vi "Material-PassFail-LineN.vi"(8 "error in (no error)":errorcluster, 10 "Line?":i32, 11 "Material-RunTest in":refnum<class "Material-RunTest.lvclass">) -> (0 "error out":errorcluster, 3 "Material-RunTest out":refnum<class "Material-RunTest.lvclass">)   [LabVIEW 2013, in "Material-RunTest.lvclass"]
uses:
  Material-RunTest.lvclass
  Material-RunTest.lvclass/Material-RunTest.ctl
  <userlib>/_MGI/1D Array/MGI Average/MGI Average (DBL[]).vi
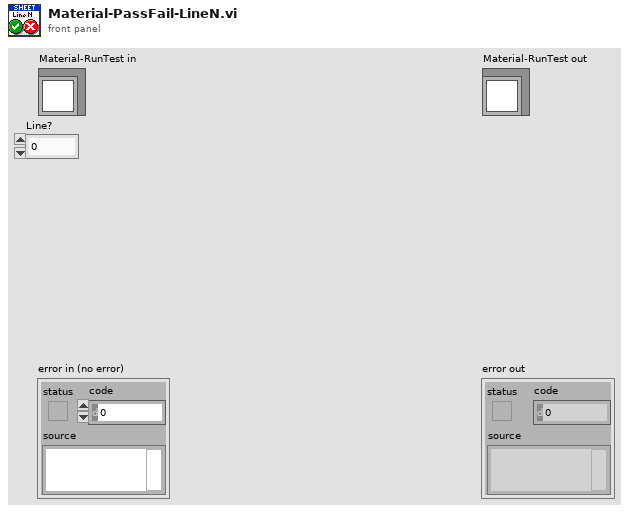
[diagram p1: front panel]
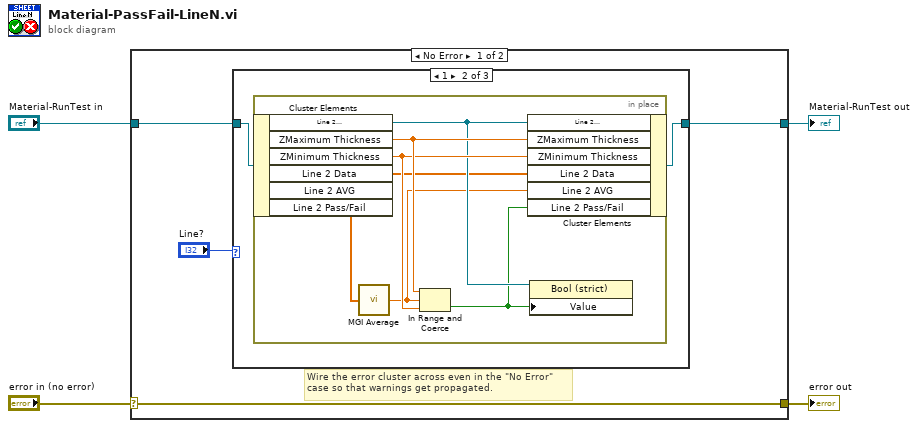
[diagram p0: block diagram]
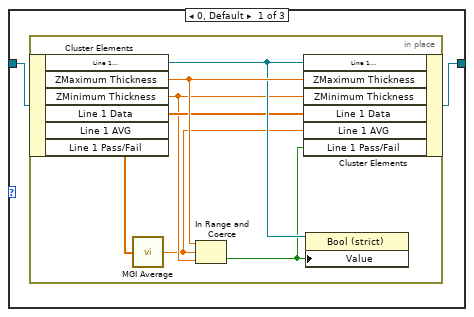
[diagram p2: hidden frame]
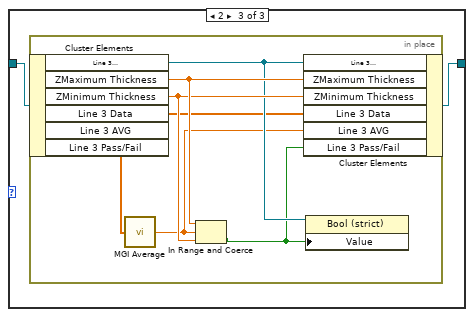
[diagram p3: hidden frame]
diagram:
  n1 = case shown="No Error" "error in (no error)" {
    selector: "error in (no error)" -> [w8 w34]
    tunnel: [w8 w34] -> w3
    tunnel: [w5 w33] -> w1
    tunnel: "Material-RunTest in" -> [w7 w33]
    frame No Error {
      # "Wire the error cluster across even in the \"No Error\"\ncase so that warnings get propagated."
      n2 = case shown="1" "Line?" {
        tunnel: w7 -> [w10 w18 w26]
        tunnel: [w9 w17 w25] -> w5
        frame 0, Default {
          n3 = in-place {
            n4 = in-place-cluster #1(w10) -> ("Line 1\ntest passed?"=w15:refnum<vi>, "ZMaximum Thickness"=w16:dbl, "ZMinimum Thickness"=w13:dbl, "Line 1 Data"=w14:dbl[])  [unwired: 2 out]
            n5 = call-poly <userlib>:"MGI Average.vi"("Double[]"=w14) -> ("Average"=w12:dbl)  [unwired: 1 in]
            n6 = In Range and Coerce(upper limit=w16, x=w12, lower limit=w13) -> (In Range?=w11:bool)  [unwired: 1 out]
            n7 = in-place-cluster #1("Line 1\ntest passed?"=w15, "ZMaximum Thickness"=w16, "ZMinimum Thickness"=w13, "Line 1 Data"=w14, "Line 1 AVG"=w12, "Line 1 Pass/Fail"=w11) -> (w9:refnum<class "Material-RunTest.lvclass">)
            n8 = property class="Bool (strict)"(reference=w15, "Value"=w11) -> ()  [unwired: 1 in, 2 out]
          }
        }
        frame 1 {
          n9 = in-place {
            n10 = in-place-cluster #2(w18) -> ("Line 2\ntest passed?"=w22:refnum<vi>, "ZMaximum Thickness"=w24:dbl, "ZMinimum Thickness"=w23:dbl, "Line 2 Data"=w21:dbl[])  [unwired: 2 out]
            n11 = call-poly <userlib>:"MGI Average.vi"("Double[]"=w21) -> ("Average"=w19:dbl)  [unwired: 1 in]
            n12 = In Range and Coerce(upper limit=w24, x=w19, lower limit=w23) -> (In Range?=w20:bool)  [unwired: 1 out]
            n13 = in-place-cluster #2("Line 2\ntest passed?"=w22, "ZMaximum Thickness"=w24, "ZMinimum Thickness"=w23, "Line 2 Data"=w21, "Line 2 AVG"=w19, "Line 2 Pass/Fail"=w20) -> (w17:refnum<class "Material-RunTest.lvclass">)
            n14 = property class="Bool (strict)"(reference=w22, "Value"=w20) -> ()  [unwired: 1 in, 2 out]
          }
        }
        frame 2 {
          n15 = in-place {
            n16 = in-place-cluster #3(w26) -> ("Line 3\ntest passed?"=w30:refnum<vi>, "ZMaximum Thickness"=w32:dbl, "ZMinimum Thickness"=w31:dbl, "Line 3 Data"=w29:dbl[])  [unwired: 2 out]
            n17 = call-poly <userlib>:"MGI Average.vi"("Double[]"=w29) -> ("Average"=w28:dbl)  [unwired: 1 in]
            n18 = In Range and Coerce(upper limit=w32, x=w28, lower limit=w31) -> (In Range?=w27:bool)  [unwired: 1 out]
            n19 = in-place-cluster #3("Line 3\ntest passed?"=w30, "ZMaximum Thickness"=w32, "ZMinimum Thickness"=w31, "Line 3 Data"=w29, "Line 3 AVG"=w28, "Line 3 Pass/Fail"=w27) -> (w25:refnum<class "Material-RunTest.lvclass">)
            n20 = property class="Bool (strict)"(reference=w30, "Value"=w27) -> ()  [unwired: 1 in, 2 out]
          }
        }
      }
    }
    frame Error {
    }
  }
  "error out" <- w3
  "Material-RunTest out" <- w1
